vi "prototype.vi"(8 "error in (no error)":errorcluster, 11 "Wash Options":T1) -> (0 "error out":errorcluster, 3 "Array":string[](array[string]))   [LabVIEW 2020]
uses:
  controls/WashOptions.ctl
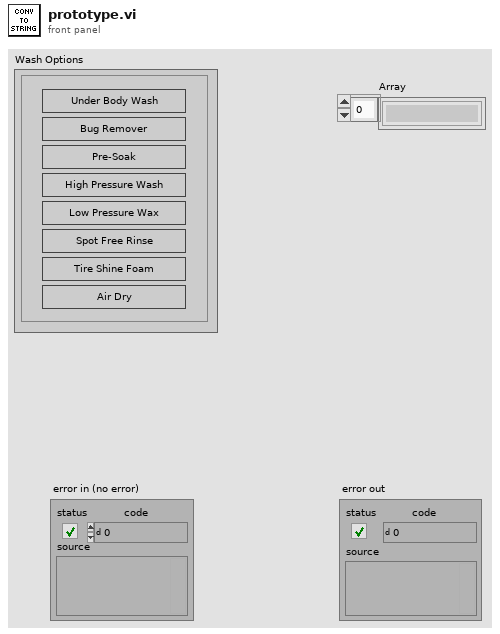
[diagram p1: front panel]
types:
  T1 = typedef "WashOptions.ctl" = cluster{"Bug Remover":bool, "Low Pressure Wax":bool, "High Pressure Wash":bool, "Pre-Soak":bool, "Spot Free Rinse":bool, "Air Dry":bool, "Under Body Wash":bool, "Tire Shine Foam":bool}
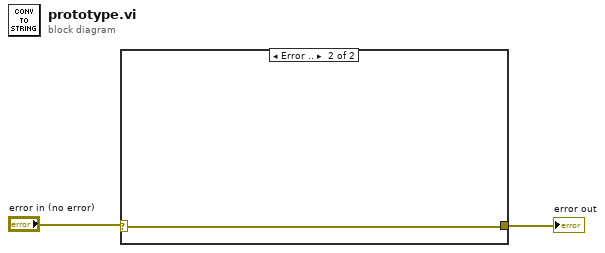
[diagram p0: block diagram]
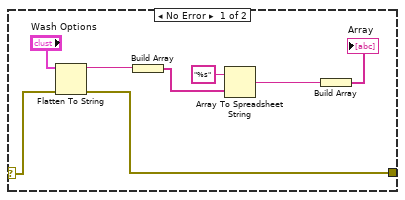
[diagram p2: hidden frame]
diagram:
  n1 = case shown="Error .." "error in (no error)" {
    selector: "error in (no error)" -> [w9 w11]
    tunnel: [w8 w11] -> w1
    frame No Error {
      n2 = Flatten To String(anything="Wash Options", error in (no error)=w9) -> (data string=w7:string, error out=w8:errorcluster)  [unwired: 2 in, 1 out]
      n3 = Build Array(w7) -> (w6:string[])
      n4 = Array To Spreadsheet String(array=w6, 3:"%s" ("format string")) -> (spreadsheet string=w5:string)  [unwired: 1 in]
      n5 = Build Array(w5) -> (→"Array":string[])
    }
    frame Error {
    }
  }
  "error out" <- w1
